vi "Get Default Values From Type Def.vi"(8 "error in (no error)":errorcluster, 11 "Type Def":variant) -> (0 "error out":errorcluster, 3 "Default Values":variant)   [LabVIEW 2020, in "MeasurementTemplate_server.lvlib"]
uses:
  MeasurementTemplate_server.lvlib
  <vilib>/Utility/Data Type/NI_Data Type.lvlib
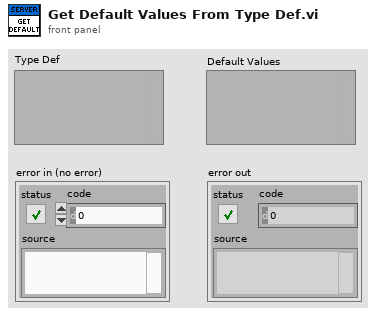
[diagram p1: front panel]
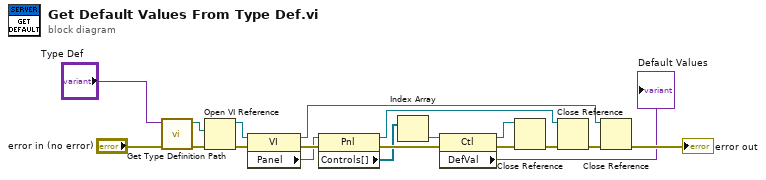
[diagram p0: block diagram]
diagram:
  n1 = call <vilib>:"Get Type Definition Path.vi"("error in (no error)"="error in (no error)", "variant"="Type Def") -> ("error out"=w15:errorcluster, "type definition path"=w4:path)  [unwired: 8 in]
  n2 = Open VI Reference(vi path=w4, error in (no error)=w15) -> (vi reference=w5:refnum<vi>, error out=w14:errorcluster)  [unwired: 4 in]
  n3 = property class="VI"(reference=w5, error in=w14) -> (reference out=w10:refnum<vi>, error out=w13:errorcluster, "Panel"=w6:refnum<vi>)
  n4 = property class="Pnl"(reference=w6, error in=w13) -> (reference out=w9:refnum<vi>, error out=w17:errorcluster, "Controls[]"=w7:refnum<vi>[])
  n5 = Index Array(array=w7) -> (element=w18:refnum<vi>)  [unwired: 1 in]
  n6 = property class="Ctl"(reference=w18, error in=w17) -> (reference out=w8:refnum<vi>, error out=w19:errorcluster, "DefVal"=→"Default Values":variant)
  n7 = Close Reference(reference=w8, error in (no error)=w19) -> (error out=w12:errorcluster)
  n8 = Close Reference(reference=w9, error in (no error)=w12) -> (error out=w11:errorcluster)
  n9 = Close Reference(reference=w10, error in (no error)=w11) -> (error out=→"error out":errorcluster)
